vi "main.vi"() -> ()   [LabVIEW 2019]
uses:
  <vilib>/vision/NI_Vision_Development_Module.lvlib
panel:
  in  "K - constant specific for stereo rig setup (distance = K / disparity)":i32=75000
  out "Right cam":T1(plugin-control)
  out "Left cam":T1(plugin-control)
  out "Object distances":cluster{string, dbl}[](array[cluster])
  in  "Stop (F)":bool
  out "Total delay (ms)":sgl
  out "Loop count":i32
  # "Overview: This VI performes object detection, distance calculation and displays the results.\n\nRequirements: LabVIEW Full Development System, NI-IMAQdx, Vision Development Module, YOLOv4 in TF\n\nWorkflow: \n1) Open block diagram and                                                                                  configure Vision Acquisition Express VI's for your cameras\n2) Set constant K\n3) Run the VI"
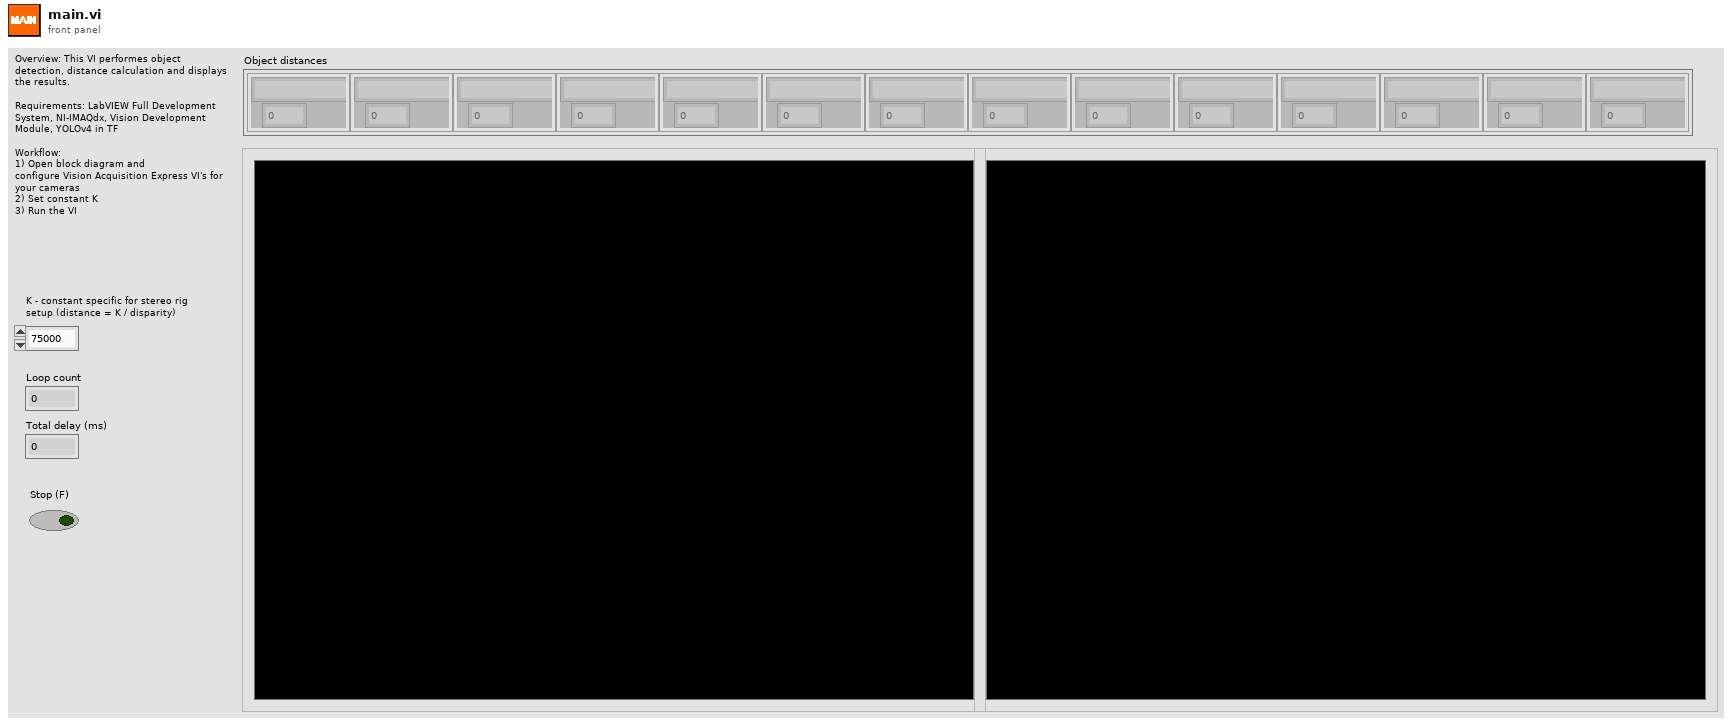
[diagram p1: front panel]
types:
  T1 = typedef "IMAQ Image.ctl" = refnum<image>
  T2 = typedef "Image Type" = u32
  T3 = cluster{"New Image":T1, "New Image":T1, "New Image":T1, "New Image":T1, "New Image":T1, "New Image":T1, "New Image":T1, "New Image":T1}
  T4 = typedef "IMAQ Binocular Stereo Session.ctl" = refnum<k1>
  T5 = cluster{"Desired Font (Application)":enum16{"User-specified Font", "Application Font", "System Font", "Dialog Font"}, "[User-specified Font]":cluster{"Font Name":string, "Size":i16, "Strikeout?":bool, "Italic?":bool, "Underline?":bool, "Outline?":bool, "Shadow?":bool, "Bold?":bool, "Rotation Angle":dbl}, "Horizontal Alignment":i16, "Vertical Alignment":i16}
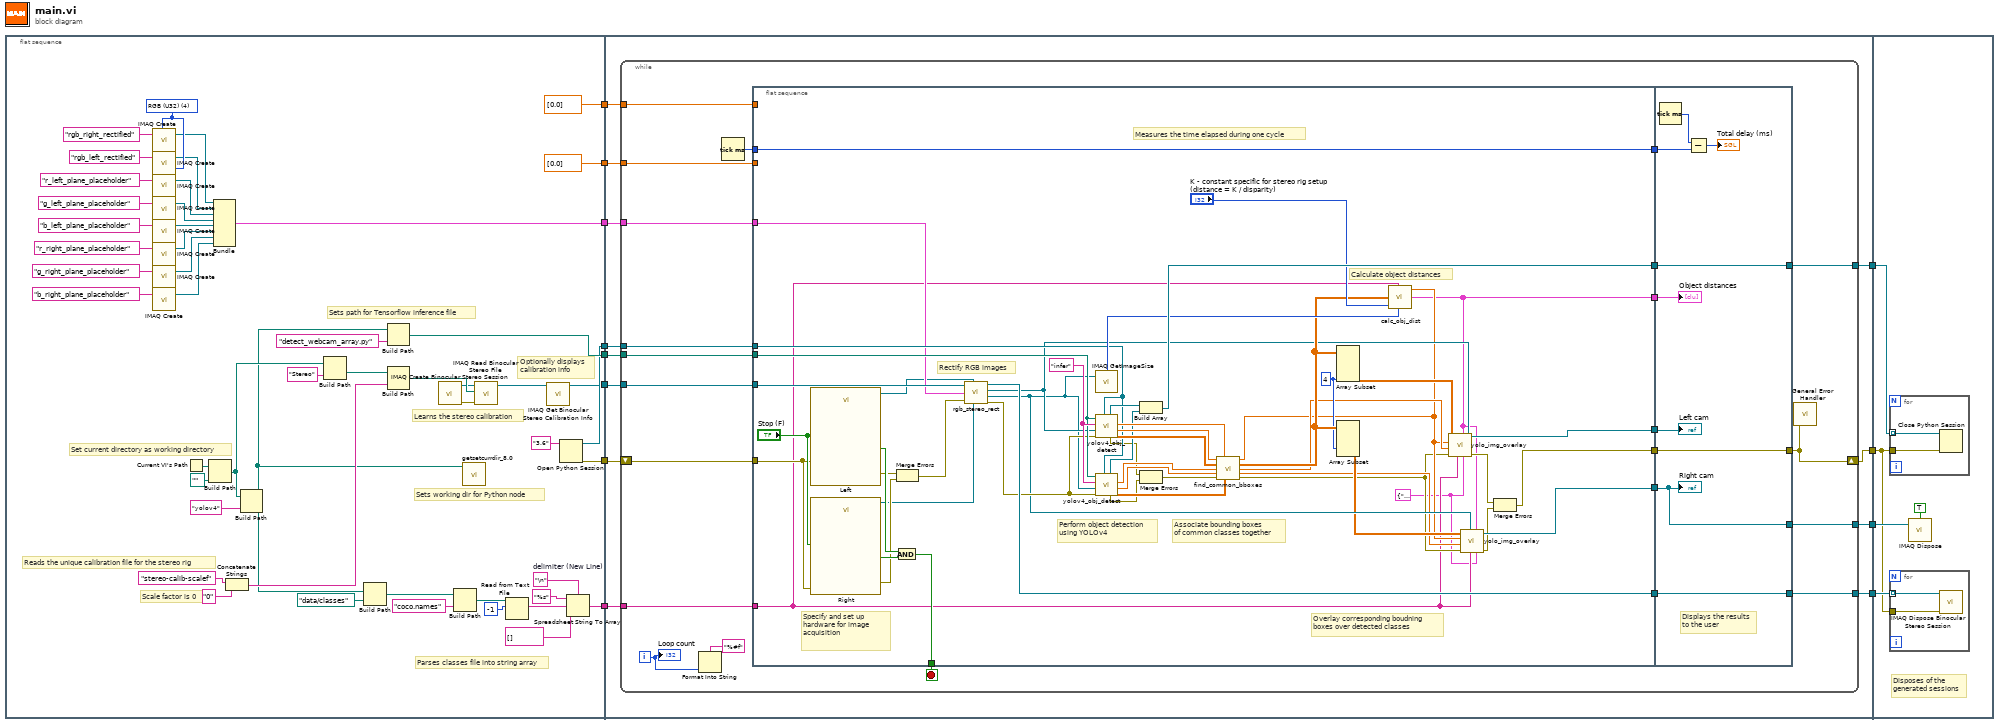
[diagram p0: block diagram]
diagram:
  n1 = flat-sequence {
    tunnel: [w44] -> w9
    tunnel: [w62] -> w8
    tunnel: [w45] -> w7
    tunnel: [dbl[] [0.0]] -> w6
    tunnel: [dbl[] [0.0]] -> w5
    tunnel: [w51] -> w4
    tunnel: [w41] -> w3
    tunnel: [w13] -> w1
    tunnel: w9 -> [w74]
    tunnel: w8 -> [w73]
    tunnel: w7 -> [w72]
    tunnel: w6 -> [w70]
    tunnel: w5 -> [w71]
    tunnel: w4 -> [w69]
    tunnel: w3 -> [w66]
    tunnel: [w68] -> w12
    tunnel: [w67] -> w11
    tunnel: [w65] -> w10
    tunnel: [w64] -> w2
    tunnel: w1 -> [w63]
    tunnel: w12 -> [w160]
    tunnel: w11 -> [w157]
    tunnel: w10 -> [w161]
    tunnel: w2 -> [w159]
    frame #0 {
      w22 = T2 4 items=["Grayscale (U8)", "Grayscale (I16)", "Grayscale (SGL)", "Complex (CSG)", "RGB (U32)", "HSL (U32)", "RGB (U64)", "Grayscale (U16)"] ("Image Type")
      w56 = "\n"  # delimiter (New Line)
      # "Scale factor is 0"
      # "Sets working dir for Python node"
      # "Optionally displays\ncalibration info"
      # "Learns the stereo calibration"
      # "Parses classes file into string array"
      # "Sets path for Tensorflow inference file"
      # "Reads the unique calibration file for the stereo rig"
      # "Set current directory as working directory"
      n2 = call "IMAQ Create"("Image Name"="rgb_right_rectified", "Image Type"=w22) -> ("New Image"=w21:T1)  [unwired: 3 in, 1 out]
      n3 = call "IMAQ Create"("Image Name"="rgb_left_rectified", "Image Type"=w22) -> ("New Image"=w20:T1)  [unwired: 3 in, 1 out]
      n4 = call "IMAQ Create"("Image Name"="r_left_plane_placeholder") -> ("New Image"=w19:T1)  [unwired: 4 in, 1 out]
      n5 = call "IMAQ Create"("Image Name"="g_left_plane_placeholder") -> ("New Image"=w18:T1)  [unwired: 4 in, 1 out]
      n6 = call "IMAQ Create"("Image Name"="b_left_plane_placeholder") -> ("New Image"=w17:T1)  [unwired: 4 in, 1 out]
      n7 = call "IMAQ Create"("Image Name"="r_right_plane_placeholder") -> ("New Image"=w14:T1)  [unwired: 4 in, 1 out]
      n8 = call "IMAQ Create"("Image Name"="g_right_plane_placeholder") -> ("New Image"=w15:T1)  [unwired: 4 in, 1 out]
      n9 = call "IMAQ Create"("Image Name"="b_right_plane_placeholder") -> ("New Image"=w16:T1)  [unwired: 4 in, 1 out]
      n10 = Current VI's Path() -> (path=w33:path)
      n11 = Build Path(base path=w33, name or relative path=path ".." ("Set Directory in")) -> (appended path=w35:path)
      n12 = Bundle("New Image"=w21, "New Image"=w20, "New Image"=w19, "New Image"=w18, "New Image"=w17, "New Image"=w14, "New Image"=w15, "New Image"=w16) -> (w13:T3)  [unwired: 1 in]
      n13 = Concatenate Strings("stereo-calib-scalef" ("name or relative path"), "0" ("string")) -> (w39:string)
      n14 = Build Path(base path=w35, name or relative path="yolov4") -> (appended path=w32:path)
      n15 = Build Path(base path=w35, name or relative path="Stereo") -> (appended path=w36:path)
      n16 = Build Path(base path=w32, name or relative path=path "data/classes" ("Set Directory in")) -> (appended path=w47:path)
      n17 = Build Path(base path=w32, name or relative path="detect_webcam_array.py") -> (appended path=w62:path)
      n18 = Build Path(base path=w36, name or relative path=w39) -> (appended path=w50:path)
      n19 = call "IMAQ Create Binocular Stereo Session"() -> ("error out"=w49:errorcluster, "Binocular Stereo Session Out"=w48:T4)  [unwired: 10 in]
      n20 = Build Path(base path=w47, name or relative path="coco.names") -> (appended path=w57:path)
      n21 = call "getsetcurrdir_8.0.vi"("Set Directory in"=w32) -> ()  [unwired: 10 in, 1 out]
      n22 = call "IMAQ Read Binocular Stereo File"("error in (no error)"=w49, "File Path"=w50, "Binocular Stereo Session (optional)"=w48) -> ("Binocular Stereo Session"=w42:T4)  [unwired: 6 in, 2 out]
      n23 = Read from Text File(file (use dialog)=w57, count=-1) -> (text=w52:string)  [unwired: 2 in, 3 out]
      n24 = call "IMAQ Get Binocular Stereo Calibration Info"("Binocular Stereo Session"=w42) -> ("Binocular Stereo Session (dup)"=w41:T4)  [unwired: 6 in, 8 out]
      n25 = Open Python Session(python version="3.6" ("Python version")) -> (session out=w44:refnum<k35>, error out=w45:errorcluster)  [unwired: 2 in]
      n26 = Spreadsheet String To Array(delimiter (Tab)=w56, format string="%s", spreadsheet string=w52, array type (2D Dbl)=string[] [] ("constant that tells LV to convert into a string arrray")) -> (array=w51:string[])
    }
    frame #1 {
      n27 = while {
        tunnel: w73 -> [w96]
        tunnel: w71 -> [w94]
        tunnel: w70 -> [w93]
        tunnel: w69 -> [w92]
        shift-right: [w78] -> w67
        shift-left: w72 -> [w95]
        tunnel: w66 -> [w89]
        tunnel: [w88] -> w65
        tunnel: w74 -> [w97]
        tunnel: [w91] -> w68
        tunnel: [w80] -> w64
        tunnel: w63 -> [w75]
        i -> [w82]
        stop <- w90 stop-if-true
        n28 = Format Into String(format string="%#f", w82) -> ()  [unwired: 2 in, 2 out]
        n29 = Tick Count (ms)() -> (millisecond timer value=w77:u32)
        n30 = flat-sequence {
          tunnel: [w147] -> w87
          tunnel: [w136] -> w86
          tunnel: [w120] -> w85
          tunnel: [w109] -> w84
          tunnel: [w106] -> w81
          tunnel: [w99] -> w79
          tunnel: w89 -> [w118]
          tunnel: [w126] -> w90
          tunnel: w92 -> [w101]
          tunnel: w93 -> [_]
          tunnel: w94 -> [_]
          tunnel: w95 -> [w124]
          tunnel: w96 -> [w132]
          tunnel: w97 -> [w129]
          tunnel: w77 -> [w122]
          tunnel: [w122] -> w76
          tunnel: w75 -> [w116]
          tunnel: w87 -> [w156]
          tunnel: w86 -> [w155]
          tunnel: w85 -> [w154]
          tunnel: w84 -> [w152]
          tunnel: w81 -> [w151]
          tunnel: [w156] -> w91
          tunnel: [w155] -> w78
          tunnel: [w154] -> w88
          tunnel: [w151] -> w80
          tunnel: w79 -> [w153]
          tunnel: w76 -> [w149]
          frame #0 {
            w113 = 4 ("length")
            w133 = "infer" ("Function name")
            w100 = T5 {"Desired Font (Application)"=enum."User-specified Font", "[User-specified Font]"={"Font Name"="", "Size"=20, "Strikeout?"=FALSE, "Italic?"=FALSE, "Underline?"=FALSE, "Outline?"=TRUE, "Shadow?"=FALSE, "Bold?"=TRUE, "Rotation Angle"=0.0}, "Horizontal Alignment"=0, "Vertical Alignment"=0} ("Font, Size & Style")
            # "Measures the time elapsed during one cycle"
            # "Calculate object distances"
            # "Overlay corresponding boudning\nboxes over detected classes"
            # "Associate bounding boxes\nof common classes together"
            # "Perform object detection\nusing YOLOv4"
            # "Rectify RGB images"
            # "Specify and set up hardware for image acquisition"
            n31 = call "Left"("Stop (F)"="Stop (F)", "error in"=w124) -> ("Image Out"=w115:T1, "Stopped"=w134:bool, "error out"=w123:errorcluster)  [unwired: 23 in]
            n32 = call "Right"("Stop (F)"="Stop (F)", "error in"=w124) -> ("Image Out"=w114:T1, "Stopped"=w135:bool, "error out"=w121:errorcluster)  [unwired: 23 in]
            n33 = And(x=w134, y=w135) -> (x .and. y?=w126:bool)
            n34 = Merge Errors(w123, w121) -> (w117:errorcluster)
            n35 = call "rgb_stereo_rect.vi"("Binocular Stereo Session (dup)"=w118, "Left image"=w115, "Input images"=w116, "error in (no error)"=w117, "Right image"=w114) -> ("Stereo session array (dup)"=w120:T4[], "Left rect image out"=w112:T1, "Right rect image out"=w107:T1, "error IO"=w119:errorcluster)
            n36 = call "IMAQ GetImageSize"("Image"=w107) -> ("X Resolution"=w145:i32)  [unwired: 3 in, 2 out]
            n37 = call "yolov4_obj_detect.vi"("Python session in"=w129, "error in (no error)"=w119, "Image Src"=w112, "Function name"=w133, "Module path"=w132) -> ("BBoxes [y_min, x_min, y_max, x_max]"=w142:dbl[][], "Scores"=w143:dbl[], "Numbered classes"=w144:dbl[], "error out"=w127:errorcluster, "Python session out"=w131:refnum<k35>)  [unwired: 1 in, 1 out]
            n38 = call "yolov4_obj_detect.vi"("Python session in"=w129, "error in (no error)"=w119, "Image Src"=w107, "Function name"=w133, "Module path"=w132) -> ("BBoxes [y_min, x_min, y_max, x_max]"=w139:dbl[][], "Scores"=w140:dbl[], "Numbered classes"=w141:dbl[], "error out"=w128:errorcluster, "Python session out"=w130:refnum<k35>)  [unwired: 1 in, 1 out]
            n39 = Build Array(w131, w130) -> (w147:refnum<k35>[])
            n40 = Merge Errors(w127, w128) -> (w138:errorcluster)
            n41 = call "find_common_bboxes.vi"("Scores L"=w143, "Class nums L"=w144, "BBoxes L"=w142, "Class nums R"=w141, "Scores R"=w140, "error in (no error)"=w138, "BBoxes R"=w139) -> ("Common classes"=w104:dbl[], "Common bboxes [y, x]"=w137:dbl[][], "Scores L"=w110:dbl[], "Scores R"=w103:dbl[], "error out"=w102:errorcluster)  [unwired: 4 in]
            n42 = Array Subset(array=w137, length (col)=w113) -> (w111:dbl[][])  [unwired: 3 in]
            n43 = Array Subset(array=w137, index (col)=w113) -> (w105:dbl[][])  [unwired: 3 in]
            n44 = call "calc_obj_dist.vi"("Common classes"=w104, "Class names"=w101, "Common bboxes"=w137, "K constant"="K - constant specific for stereo rig setup (distance = K / disparity)", "X Resolution"=w145) -> ("Object distances"=w99:cluster{string, dbl}[])
            n45 = call "yolo_img_overlay.vi"("Font, Size & Style"=w100, "Distances"=w99, "Class names"=w101, "Input image"=w112, "error in (no error)"=w102, "Scores"=w110, "Numbered classes"=w104, "BBoxes [y_min, x_min, y_max, x_max]"=w111) -> ("error out"=w108:errorcluster, "Overlaid image"=w109:T1)  [unwired: 1 in, 1 out]
            n46 = call "yolo_img_overlay.vi"("Font, Size & Style"=w100, "Distances"=w99, "Class names"=w101, "Input image"=w107, "error in (no error)"=w102, "Scores"=w103, "Numbered classes"=w104, "BBoxes [y_min, x_min, y_max, x_max]"=w105) -> ("error out"=w98:errorcluster, "Overlaid image"=w106:T1)  [unwired: 1 in, 1 out]
            n47 = Merge Errors(w108, w98) -> (w136:errorcluster)
          }
          frame #1 {
            # "Displays the results\nto the user"
            n48 = Tick Count (ms)() -> (millisecond timer value=w150:u32)
            n49 = Subtract(x=w150, y=w149) -> (x-y=→"Total delay (ms)":u32)
            "Object distances" <- w153
            "Left cam" <- w152
            "Right cam" <- w151
          }
        }
        n50 = call <vilib>:"General Error Handler.vi"("error in (no error)"=w78) -> ()  [unwired: 10 in, 5 out]
        "Loop count" <- w82
      }
    }
    frame #2 {
      # "Disposes of the \ngenerated sessions"
      n51 = for {
        tunnel: w160 -> [w165] mode=indexing
        tunnel: w157 -> [w164]
        n52 = Close Python Session(session in=w165, error in=w164) -> ()  [unwired: 1 out]
      }
      n53 = for {
        tunnel: w161 -> [w163] mode=indexing
        tunnel: w157 -> [w162]
        n54 = call "IMAQ Dispose Binocular Stereo Session"("error in (no error)"=w162, "Binocular Stereo Session"=w163) -> ()  [unwired: 9 in, 1 out]
      }
      n55 = call "IMAQ Dispose"("All Images? (No)"=TRUE, "Image"=w159) -> ()  [unwired: 4 in, 1 out]
    }
  }
